vi "Joystick Drive.vi"(0 "Joystick Drive":T2) -> (1 "Strafe":dbl, 2 "Forward/Backward":dbl, 3 "Turn":dbl)   [LabVIEW 2013]
uses:
  <vilib>/Rock Robotics/WPI/Joystick/WPI_JoystickButtonState.ctl
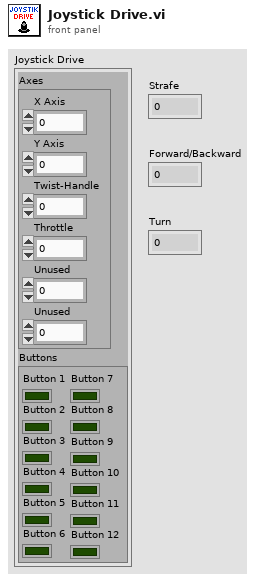
[diagram p1: front panel]
types:
  T1 = typedef "WPI_JoystickButtonState.ctl" = cluster{"Button 1":bool, "Button 2":bool, "Button 3":bool, "Button 4":bool, "Button 5":bool, "Button 6":bool, "Button 7":bool, "Button 8":bool, "Button 9":bool, "Button 10":bool, "Button 11":bool, "Button 12":bool}
  T2 = cluster{"Axes":cluster{"X Axis":dbl, "Y Axis":dbl, "Twist-Handle":dbl, "Throttle":dbl, "Unused":dbl, "Unused":dbl}, "Buttons":T1}
  T3 = cluster{"X Axis":dbl, "Y Axis":dbl, "Twist-Handle":dbl, "Throttle":dbl, "Unused":dbl, "Unused":dbl}
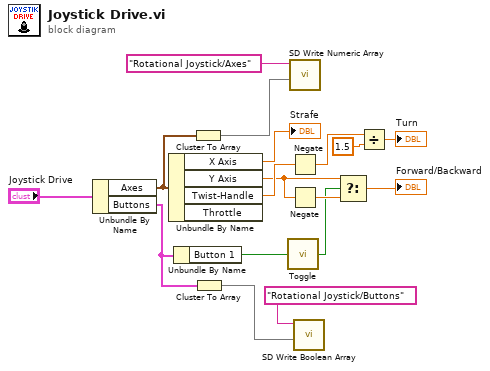
[diagram p0: block diagram]
diagram:
  n1 = Unbundle By Name("Joystick Drive") -> ("Axes"=w14:T3, "Buttons"=w6:T1)
  n2 = Unbundle By Name(w14) -> ("X Axis"=→"Strafe":dbl, "Y Axis"=w4:dbl, "Twist-Handle"=w12:dbl)  [unwired: 1 out]
  n3 = Unbundle By Name(w6) -> ("Button 1"=w3:bool)
  n4 = Cluster To Array(cluster=w14) -> (array=w15:dbl[])
  n5 = Cluster To Array(cluster=w6) -> (array=w7:bool[])
  n6 = call "Toggle.vi"("Input"=w3) -> ("Latched"=w2:bool)
  n7 = call <vilib>:"SD Write Numeric Array.vi"("Numeric Array"=w15, "Name"="Rotational Joystick/Axes") -> ()  [unwired: 8 in, 2 out]
  n8 = Negate(x=w12) -> (-x=w10:dbl)
  n9 = Negate(x=w4) -> (-x=w5:dbl)
  n10 = call <vilib>:"SD Write Boolean Array.vi"("Boolean Array"=w7, "Name"="Rotational Joystick/Buttons") -> ()  [unwired: 8 in, 2 out]
  n11 = Select(t=w4, s=w2, f=w5) -> (s? t:f=→"Forward/Backward":dbl)
  n12 = Divide(x=w10, y=1.5) -> (x/y=→"Turn":dbl)
